vi "pos_gen.vi"(11 "theta":dbl) -> (3 "x_d":dbl)   [LabVIEW 2013]
uses:
  <vilib>/Simulation/Implementation/XNodeFramework/SimXNode/SimX.xnode
  amplitud_lookup.vi
  <vilib>/Simulation/Implementation/Shared/SIMSCR Execution Mode.ctl
  <vilib>/Simulation/Scripting/Companion Diagram/SimConfigNode/_simSolvers.ctl
  <vilib>/Simulation/Scripting/Companion Diagram/SimConfigNode/SimParams.ctl
  <vilib>/Simulation/Scripting/Companion Diagram/SimConfigNode/SimDog.xnode
  <vilib>/Simulation/Implementation/Shared/SIM Bundle Sim Info.vi
  <vilib>/Simulation/Implementation/Shared/SIM Unbundle Sim Info.vi
  <vilib>/Simulation/Implementation/Shared/NILVSim_FinalizeModel.vi
  <vilib>/Simulation/Implementation/Shared/NILVSim_GetModelError.vi
  <vilib>/Simulation/Implementation/Shared/NILVSim_Initialize.vi
  <vilib>/Simulation/Utility/Implementation/NILVSim Get Time and IsAcceptedStep.vi
  <vilib>/Simulation/Implementation/Shared/NILVSim_Manager.vi
  <vilib>/Simulation/Implementation/Shared/NI_SIM_Implementation.lvlib
  <vilib>/Simulation/Implementation/Shared/NILVSIM_BeginStep.vi
  <vilib>/Simulation/Param Hierarchy/Typedefs/SIMPH Param Control Actions.ctl
  <vilib>/Simulation/Implementation/Shared/NILVSim_ParamChanged.vi
  <vilib>/Utility/error.llb/Clear Errors.vi
  <vilib>/Simulation/Implementation/Shared/SIMSH Read Queue.vi
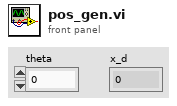
[diagram p1: front panel]
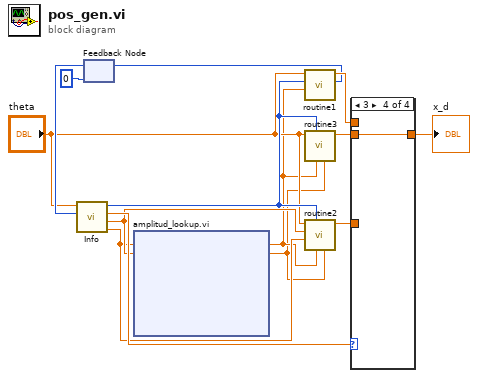
[diagram p0: block diagram]
diagram:
  n1 = feedback #1(i16 0 ("done")) -> (w9:i16)
  n2 = call "Info.vi"("done"=w9, "theta"="theta") -> ("theta_min"=w6:dbl, "theta_max"=w7:dbl, "routine"=w11:dbl, "section"=w4:i16)  [unwired: 6 in]
  n3 = xnode "amplitud_lookup.vi"("theta_min"=w6, "theta_max"=w7) -> ("amp1"=w2:dbl, "amp3"=w1:dbl)  [unwired: 2 in, 9 out]
  n4 = call "routine1.vi"("amp1"=w2, "section"=w4, "theta"="theta") -> ("done"=w8:i16, "x_d1"=w12:dbl)  [unwired: 7 in]
  n5 = feedback-in #1(w8) -> ()
  n6 = call "routine3.vi"("amp3"=w1, "amp1"=w2, "section"=w4, "theta"="theta") -> ("x_d3"=w5:dbl)  [unwired: 7 in]
  n7 = call "routine2.vi"("amp3"=w1, "amp1"=w2, "section"=w4, "theta_min"=w6, "theta_max"=w7, "theta"="theta") -> ("x_d2"=w13:dbl)  [unwired: 5 in]
  n8 = case shown="3" w11 {
    tunnel: [_ w15 w16 w17] -> w14
    tunnel: w12 -> [_ w15 _ _]
    tunnel: w13 -> [_ _ w16 _]
    tunnel: w5 -> [_ _ _ w17]
    frame 0, Default {
    }
    frame 1 {
    }
    frame 2 {
    }
    frame 3 {
    }
  }
  "x_d" <- w14
